vi "IsRefnum.vi"(8 "error in":errorcluster, 11 "CustomDataType in":refnum<class "CustomData.lvclass">) -> (0 "error out":errorcluster, 2 "IsRefnum":bool, 3 "CustomDataType out":refnum<class "CustomData.lvclass">)   [LabVIEW 2021, in "ProligentXMLGenerator.lvlib" / "CustomData.lvclass"]
doc: "Returns TRUE if the passed object is valid."
uses:
  CustomData.lvclass
  CustomData.lvclass/CustomData.ctl
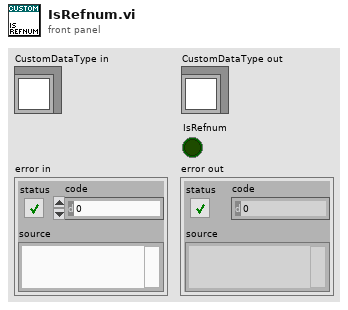
[diagram p1: front panel]
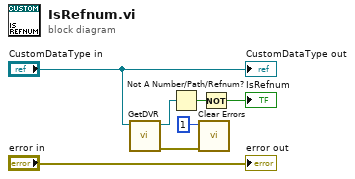
[diagram p0: block diagram]
diagram:
  n1 = call "GetDVR.vi"("CustomDataType"="CustomDataType in") -> ("error out"=w1:errorcluster, "DVRReference"=w5:refnum<data-value>)  [unwired: 9 in]
  n2 = Not A Number/Path/Refnum?(number/path/refnum=w5) -> (NaN/Path/Refnum?=w6:bool)
  n3 = call <vilib>:"Clear Errors.vi"("error in (no error)"=w1, "specific error code to clear (0: all)"=1) -> ()  [unwired: 4 in, 2 out]
  n4 = Not(x=w6) -> (.not. x?=→"IsRefnum":bool)
  "error out" <- "error in"
  "CustomDataType out" <- "CustomDataType in"
